vi "GDS_MO_SetEnergy170615.vi"(11 "AEnergy":dbl=8.0) -> ()   [LabVIEW 2015]
uses:
  C/Program Files/National Instruments/LabVIEW 2015/user.lib/caLab/Private/Get_PV-1D.vi
  C/Program Files/National Instruments/LabVIEW 2015/user.lib/caLab/Private/Put_DBL_PV.vi
panel:
  out "SPEC:BUSY":dbl
  out "SPEC:INC":dbl
  out "retrun value":i32
  out "SPEC:ExpNumber_RV":dbl=99.0
  # "SetEnergy"
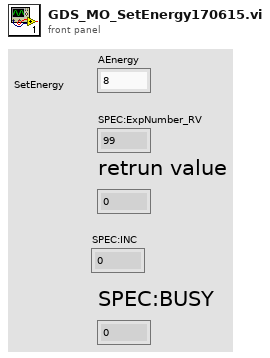
[diagram p1: front panel]
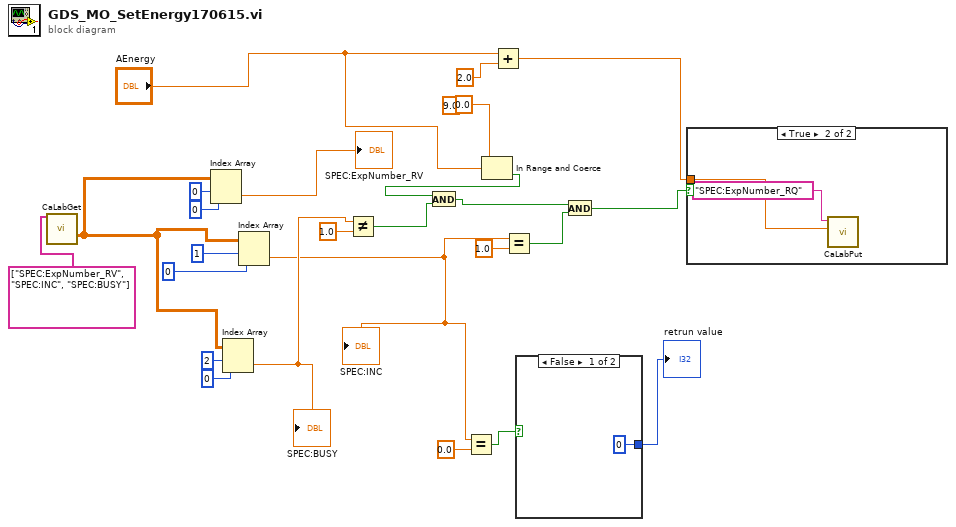
[diagram p0: block diagram]
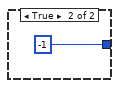
[diagram p3: hidden frame]
diagram:
  n1 = call-poly "CaLabGet.vi"("PV Names"=string[] ["SPEC:ExpNumber_RV", "SPEC:INC", "SPEC:BUSY"]) -> ("Value Array (number)"=w19:dbl[][])  [unwired: 8 in, 6 out]
  n2 = Index Array(array=w19, index (row)=0, index (col)=0 ("disabled index (col)")) -> (element=→"SPEC:ExpNumber_RV":dbl)
  n3 = Index Array(array=w19, index (row)=2, index (col)=0 ("disabled index (col)")) -> (element=w14:dbl)
  "SPEC:BUSY" <- w14
  n4 = Index Array(array=w19, index (row)=1, index (col)=0 ("disabled index (col)")) -> (element=w12:dbl)
  "SPEC:INC" <- w12
  n5 = Not Equal?(x=w14, y=1.0) -> (x != y?=w13:bool)
  n6 = Equal?(x=w12, y=0.0) -> (x = y?=w17:bool)
  n7 = In Range and Coerce(upper limit=9.0, x="AEnergy", lower limit=0.0) -> (In Range?=w1:bool)  [unwired: 1 out]
  n8 = And(x=w1, y=w13) -> (x .and. y?=w10:bool)
  n9 = Add(x="AEnergy", y=2.0) -> (x+y=w6:dbl)
  n10 = Equal?(x=w12, y=1.0) -> (x = y?=w9:bool)
  n11 = case shown="False" w17 {
    tunnel: [0 -1] -> w16
    frame False {
    }
    frame True {
    }
  }
  "retrun value" <- w16
  n12 = And(x=w10, y=w9) -> (x .and. y?=w8:bool)
  n13 = case shown="True" w8 {
    tunnel: w6 -> [_ w29]
    frame False {
    }
    frame True {
      n14 = call-poly "CaLabPut.vi"("Value"=w29, "PV Name"="SPEC:ExpNumber_RQ") -> ()  [unwired: 6 in, 4 out]
    }
  }
